vi "TestPanel.vi"() -> ()   [LabVIEW 2017, in "MenuButtons.lvlib"]
uses:
  MenuButtons.lvlib
  MenuButton/MenuButton.lvclass
  MenuButton Event Handler/MenuButton Event Handler.lvclass
panel:
  in  "SubItem2 2":bool
  in  "SubItem1 2":bool
  in  "SubItem2":bool
  in  "SubItem1":bool
  in  "Main Menu 2":bool
  in  "Main Menu1":bool
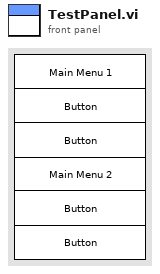
[diagram p1: front panel]
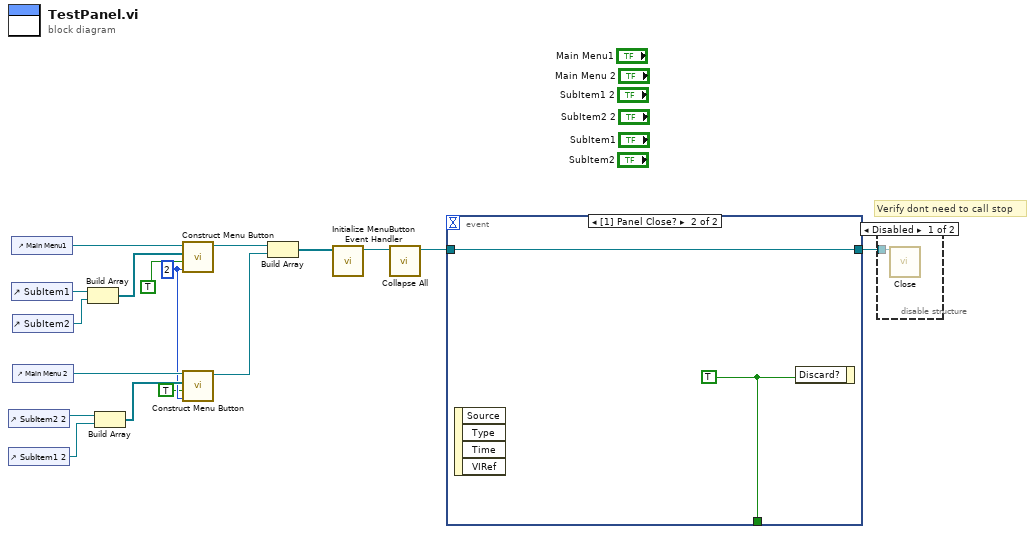
[diagram p0: block diagram]
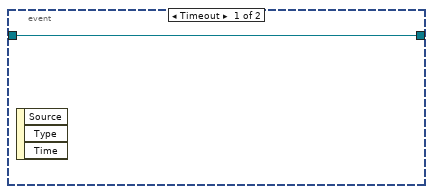
[diagram p3: hidden frame]
diagram:
  w8 = 2 ("Border Offset")
  # "Verify dont need to call stop"
  n1 = control-ref of="SubItem2 2"() -> (w12:refnum<vi>)
  n2 = control-ref of="SubItem1 2"() -> (w11:refnum<vi>)
  n3 = control-ref of="Main Menu1"() -> (w17:refnum<vi>)
  n4 = control-ref of="SubItem1"() -> (w16:refnum<vi>)
  n5 = control-ref of="SubItem2"() -> (w15:refnum<vi>)
  n6 = control-ref of="Main Menu 2"() -> (w13:refnum<vi>)
  n7 = Build Array(w16, w15) -> (w14:refnum<vi>[])
  n8 = Build Array(w12, w11) -> (w10:refnum<vi>[])
  n9 = call "Construct Menu Button.vi"("Border Offset"=w8, "Reset Bool on Value Change?"=TRUE, "Nested Item Refs"=w14, "Menu Reference"=w17) -> ("MenuButton out"=w7:refnum<class "MenuButton.lvclass">)  [unwired: 7 in]
  n10 = call "Construct Menu Button.vi"("Border Offset"=w8, "Reset Bool on Value Change?"=TRUE, "Nested Item Refs"=w10, "Menu Reference"=w13) -> ("MenuButton out"=w6:refnum<class "MenuButton.lvclass">)  [unwired: 7 in]
  n11 = Build Array(w7, w6) -> (w4:refnum<class "MenuButton.lvclass">[])
  n12 = call "Initialize MenuButton Event Handler.vi"("Menu Buttons"=w4) -> ("MenuButton Event Handler out"=w2:refnum<class "MenuButton Event Handler.lvclass">)  [unwired: 9 in, 1 out]
  n13 = call "Collapse All.vi"("MenuButton Event Handler in"=w2) -> ("MenuButton Event Handler out"=w1:refnum<class "MenuButton Event Handler.lvclass">)  [unwired: 9 in, 1 out]
  n14 = event shown="[1] Panel Close?" {
    selector: _ -> [_ _]
    dyn-events: _ -> [_ _]
    timeout: _ -> [_ _]
    tunnel: w1 -> [w18 w19]
    tunnel: [w18 w19] -> w3
    tunnel: [_ w20] -> _
    event Timeout {
      n15 = event-data() -> ()  [unwired: 1 in, 3 out]
    }
    event Panel Close? {
      w20 = TRUE
      n16 = event-data() -> ()  [unwired: 1 in, 4 out]
      n17 = event-data("Discard?"=w20) -> ()  [unwired: 1 in, 1 out]
    }
  }
  n18 = disable-structure shown="Disabled" {
    disable-tunnel: w3 -> [w21 _]
    frame Disabled {
      n19 = call "Close.vi"("MenuButton Event Handler in"=w21) -> ()  [unwired: 10 in, 1 out]
    }
    frame Enabled {
    }
  }
